vi "Close the Loop.vi"(8 "P_toolf":dbl[](array[numeric]), 9 "S_n-1f":dbl[](array[numeric]), 10 "a_(n-1)nf":dbl[](array[numeric]), 11 "Analytical Serial Arm Class in":refnum<class "NI_Robotics_Analytical Serial Arm Class.lvclass">) -> (1 "gamma_0":dbl, 2 "theta_n":dbl, 3 "Analytical Serial Arm Class out":refnum<class "NI_Robotics_Analytical Serial Arm Class.lvclass">)   [LabVIEW 2017, in "NI_Robotics_Analytical Serial Arm Class.lvclass"]
uses:
  <vilib>/robotics/Kinematics/Analytical/Generic/NI_Robotics_Analytical Serial Arm Class.lvclass
  <vilib>/Analysis/_algsub.llb/Vector Norm.vi
  <vilib>/Analysis/_algsub.llb/Real Vector Norm.vi
  <vilib>/Analysis/baseanly.llb/Dot Product.vi
  <vilib>/Analysis/baseanly.llb/Real Dot Product.vi
  <vilib>/robotics/Kinematics/Analytical/Generic/Accessors/Write S_0.vi
  <vilib>/robotics/Kinematics/Analytical/Generic/Accessors/Write alpha_n0.vi
  <vilib>/robotics/Kinematics/Analytical/Generic/Accessors/Write a_n0.vi
  <vilib>/Analysis/coordinate.llb/Cross Product.vi
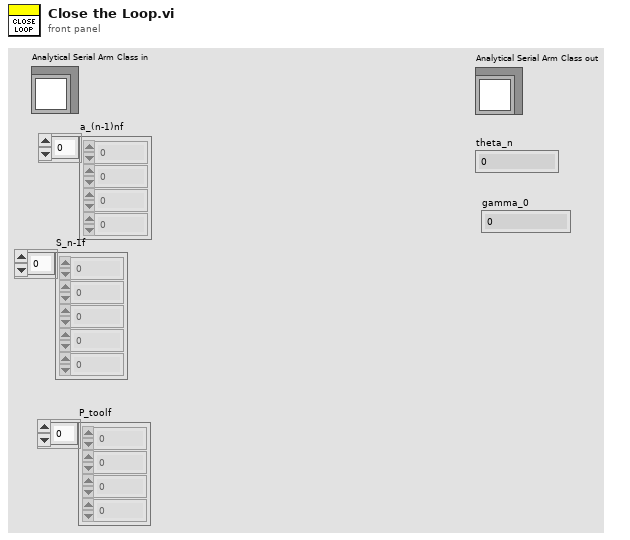
[diagram p1: front panel]
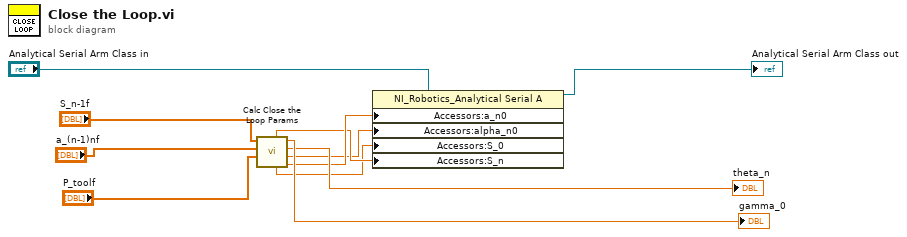
[diagram p0: block diagram]
diagram:
  n1 = call <vilib>:"Calc Close the Loop Params.vi"("P_toolf"="P_toolf", "a_67f"="a_(n-1)nf", "S_6f"="S_n-1f") -> ("a_71"=w4:dbl, "alpha_71"=w1:dbl, "theta_7"=→"theta_n":dbl, "gamma_1"=→"gamma_0":dbl, "S_1"=w2:dbl, "S_7"=w3:dbl)  [unwired: 3 in]
  n2 = property class="NI_Robotics_Analytical Serial A"(reference="Analytical Serial Arm Class in", "Accessors:a_n0"=w4, "Accessors:alpha_n0"=w1, "Accessors:S_0"=w2, "Accessors:S_n"=w3) -> (reference out=→"Analytical Serial Arm Class out":refnum<class "NI_Robotics_Analytical Serial Arm Class.lvclass">)  [unwired: 1 in, 1 out]
